vi "Test_ANN_NEW.vi"(8 "rt fifo READ":refnum<k33>, 11 "rt fifo SEND":refnum<k33>) -> (2 "Acc":dbl)   [LabVIEW 2020]
uses:
  Store Training and Testing set.vi
panel:
  out "Prediction":sgl[](array[numeric])
  out "Real":sgl[](array[numeric])
  out "good":i32
  out "total":i32
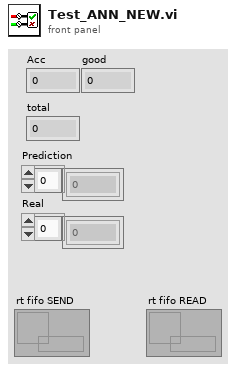
[diagram p1: front panel]
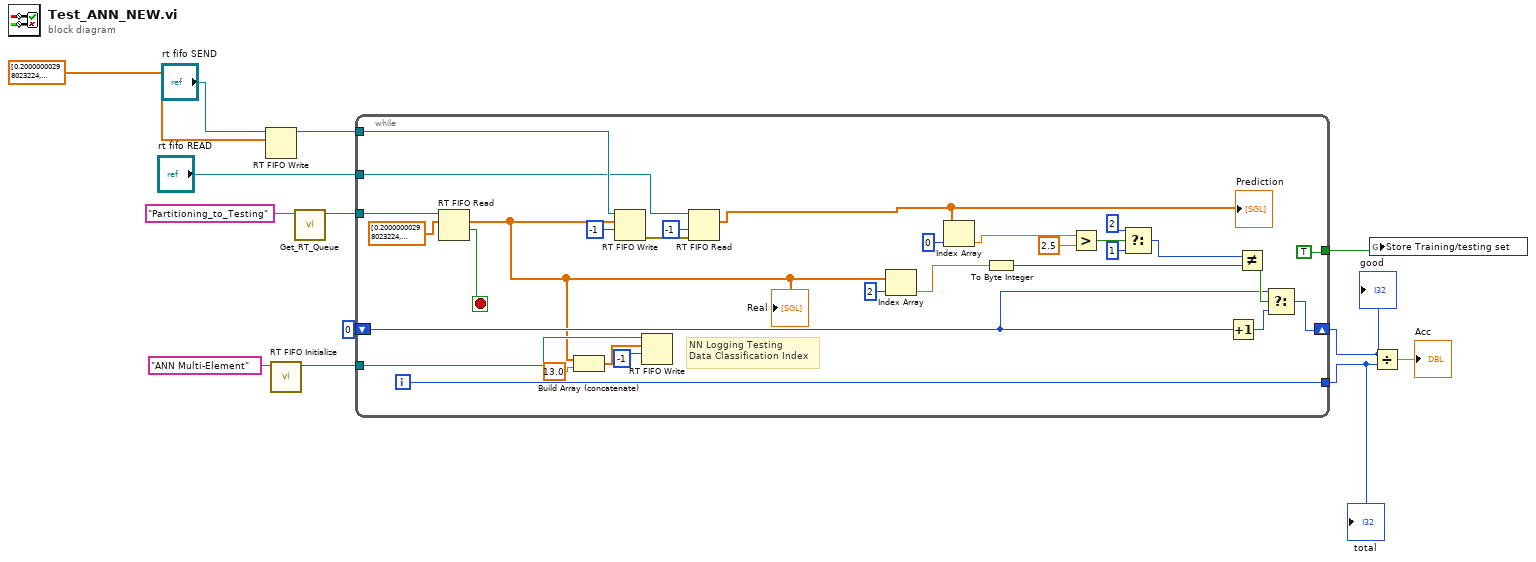
[diagram p0: block diagram]
diagram:
  n1 = RT FIFO Write(0:"rt fifo SEND", 1:sgl[] [0.2, 0.2, -1.0, 0.0, 0.0, 0.0, 0.0, 0.0] ("Data to FPGA")) -> (8:w1:refnum<k33>)  [unwired: 3 in, 3 out]
  n2 = call "RT FIFO Initialize.vi"("name (unnamed)"="ANN Multi-Element") -> ("rt fifo"=w6:refnum<k33>)  [unwired: 9 in, 1 out]
  n3 = call "Get_RT_Queue.vi"("String"="Partitioning_to_Testing") -> ("rt fifo single"=w8:refnum<k33>)  [unwired: 8 in, 2 out]
  n4 = while {
    shift-right: [w37] -> w12
    shift-left: 0 -> [w39]
    tunnel: [w41] -> w11
    tunnel: w8 -> [w36]
    tunnel: w6 -> [w23]
    tunnel: [TRUE] -> w5
    tunnel: "rt fifo READ" -> [w15]
    tunnel: w1 -> [w16]
    i -> [w41]
    stop <- w43 stop-if-true
    # "NN Logging Testing \nData Classification Index"
    n5 = RT FIFO Read(0:w36, 1:sgl[] [0.2, 0.2, -1.0, 0.0, 0.0, 0.0, 0.0, 0.0] ("Data to FPGA")) -> (9:w21:sgl[], 10:w43:bool)  [unwired: 2 in, 3 out]
    "Real" <- w21
    n6 = Build Array (concatenate)(w21, 13.0) -> (w26:dbl[])
    n7 = RT FIFO Write(0:w16, 1:w21, 2:-1 ("Timeout (ms)")) -> (11:w19:errorcluster)  [unwired: 2 in, 3 out]
    n8 = RT FIFO Write(0:w23, 1:w26, 2:-1 ("timeout in ms (0)")) -> ()  [unwired: 2 in, 4 out]
    n9 = RT FIFO Read(0:w15, 2:-1 ("timeout in ms (0)"), 3:w19) -> (9:w17:sgl[])  [unwired: 1 in, 4 out]
    "Prediction" <- w17
    n10 = Index Array(array=w21, index=2) -> (element=w34:sgl)
    n11 = Index Array(array=w17, index=0) -> (element=w32:sgl)
    n12 = To Byte Integer(number=w34) -> (8bit integer=w33:i8)
    n13 = Greater?(x=w32, y=sgl 2.5) -> (0:w30:bool)
    n14 = Select(t=i8 2, s=w30, f=i8 1) -> (s? t:f=w27:i8)
    n15 = Increment(x=w39) -> (x+1=w38:i32)
    n16 = Not Equal?(x=w27, y=w33) -> (x != y?=w40:bool)
    n17 = Select(t=w39, s=w40, f=w38) -> (s? t:f=w37:i32)
  }
  "total" <- w11
  "good" <- w12
  n18 = global write "Store Training and Testing set.vi" "Store Training/testing set"(w5) -> ()
  n19 = Divide(x=w12, y=w11) -> (x/y=→"Acc":dbl)
